vi "11c-async.vi"() -> ()   [LabVIEW 2018, in "LV2Julia_examples.lvlib"]
uses:
  LV2Julia_core/VIs/Server or client state.ctl
  LV2Julia_core/VIs/detailed error info.ctl
  LV2Julia_core/VIs/StackFrame.ctl
  LV2Julia_core/VIs/Commands.ctl
  be4745b6-8471-45fc-b8a0-8968ce92ea4b.vi
  877f6708-f4bd-42a3-8abe-32eb8c2c970e.vi
  be4745b6-8471-45fc-b8a0-8968ce92ea4b.vi/01ce1741-ea78-47f8-98ed-e79163fb1a9b.vi
  877f6708-f4bd-42a3-8abe-32eb8c2c970e.vi/896d20f1-cb1d-4420-8f1f-f93355f5adea.vi
  be4745b6-8471-45fc-b8a0-8968ce92ea4b.vi/01ce1741-ea78-47f8-98ed-e79163fb1a9b.vi/cc3cf2af-bc3b-4fb6-855b-7562c4d0bfeb.vi
  be4745b6-8471-45fc-b8a0-8968ce92ea4b.vi/01ce1741-ea78-47f8-98ed-e79163fb1a9b.vi/c77cecd8-10de-4d46-bc1c-57302a887fda.vi
  be4745b6-8471-45fc-b8a0-8968ce92ea4b.vi/01ce1741-ea78-47f8-98ed-e79163fb1a9b.vi/2cafb1dd-d397-4b79-911a-06d102936120.vi
  877f6708-f4bd-42a3-8abe-32eb8c2c970e.vi/896d20f1-cb1d-4420-8f1f-f93355f5adea.vi/9892c125-836d-426b-b144-8af50d50507b.vi
  877f6708-f4bd-42a3-8abe-32eb8c2c970e.vi/896d20f1-cb1d-4420-8f1f-f93355f5adea.vi/80aac079-9052-42cf-b2c3-c29da6bba58d.vi
  877f6708-f4bd-42a3-8abe-32eb8c2c970e.vi/896d20f1-cb1d-4420-8f1f-f93355f5adea.vi/6d5e1d21-cb4d-4981-8d16-85d9352ac501.vi
  LV2Julia_core/VIs/jl-scripts path.vi
  LV2Julia_core/VIs/check ID validity.vi
  LV2Julia_core/VIs/bindata_descr to JSON.vi
  LV2Julia_core/VIs/check cluster field names.vi
  LV2Julia_core/VIs/concat JSON.vi
  LV2Julia_core/VIs/build request.vi
  LV2Julia_core/VIs/Parse server response.vi
  LV2Julia_core/VIs/log jl exceptions.vi
  LV2Julia_examples.lvlib
  LV2Julia_core/LV2Julia_core.lvlib
panel:
  in  "Timeout (s)":dbl
  out "notif 2":bool
  out "Boolean":bool
  out "notification":bool
  in  "stop polling":bool
  out "stopping":bool
  out "done":bool
  out "ticket":i32
  in  "summands":cluster{"x":dbl, "y":dbl}={"x"=2.0, "y"=2.0}
  in  "next":bool
  out "x+y":dbl=nan
  out "detailed error info":T1
  out "current error":errorcluster
  out "final error":errorcluster
  out "short err code":u8
  in  "stop":bool
  out "ZMQ timeout":bool
  out "Julia script file path":path
  out "temporary script path":path
  out "Jl Server state":T3
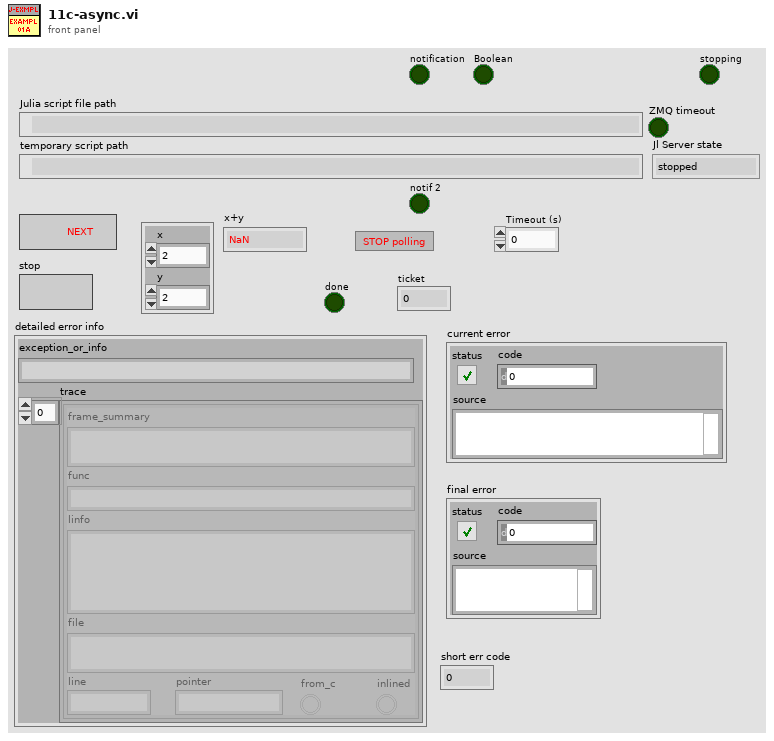
[diagram p1: front panel]
types:
  T1 = typedef "LV2Julia_core.lvlib/detailed error info.ctl" = cluster{"exception_or_info":string, "trace":T2[]}
  T2 = typedef "LV2Julia_core.lvlib/StackFrame.ctl" = cluster{"frame_summary":string, "func":string, "linfo":string, "file":string, "line":i32, "pointer":u64, "from_c":bool, "inlined":bool}
  T3 = typedef "LV2Julia_core.lvlib/Server or client state.ctl" = enum16{"stopped", "running", "unknown"}
  T4 = typedef "LV2Julia_core.lvlib/Commands.ctl" = enum16{"Start Jl-server & Init LV-client", "Send request & Get response ", "Stop Jl-server & Cleanup LV-client", "Cleanup LV-client", "Start Jl-server", "Stop Jl-server", "Init LV-Client", "Cleanup LV-Client", "(not allowed)", "Set LV Client state", "Set Jl Server state", "set ZMQ timeout", "read ZMQ timeout", "read-out state"}
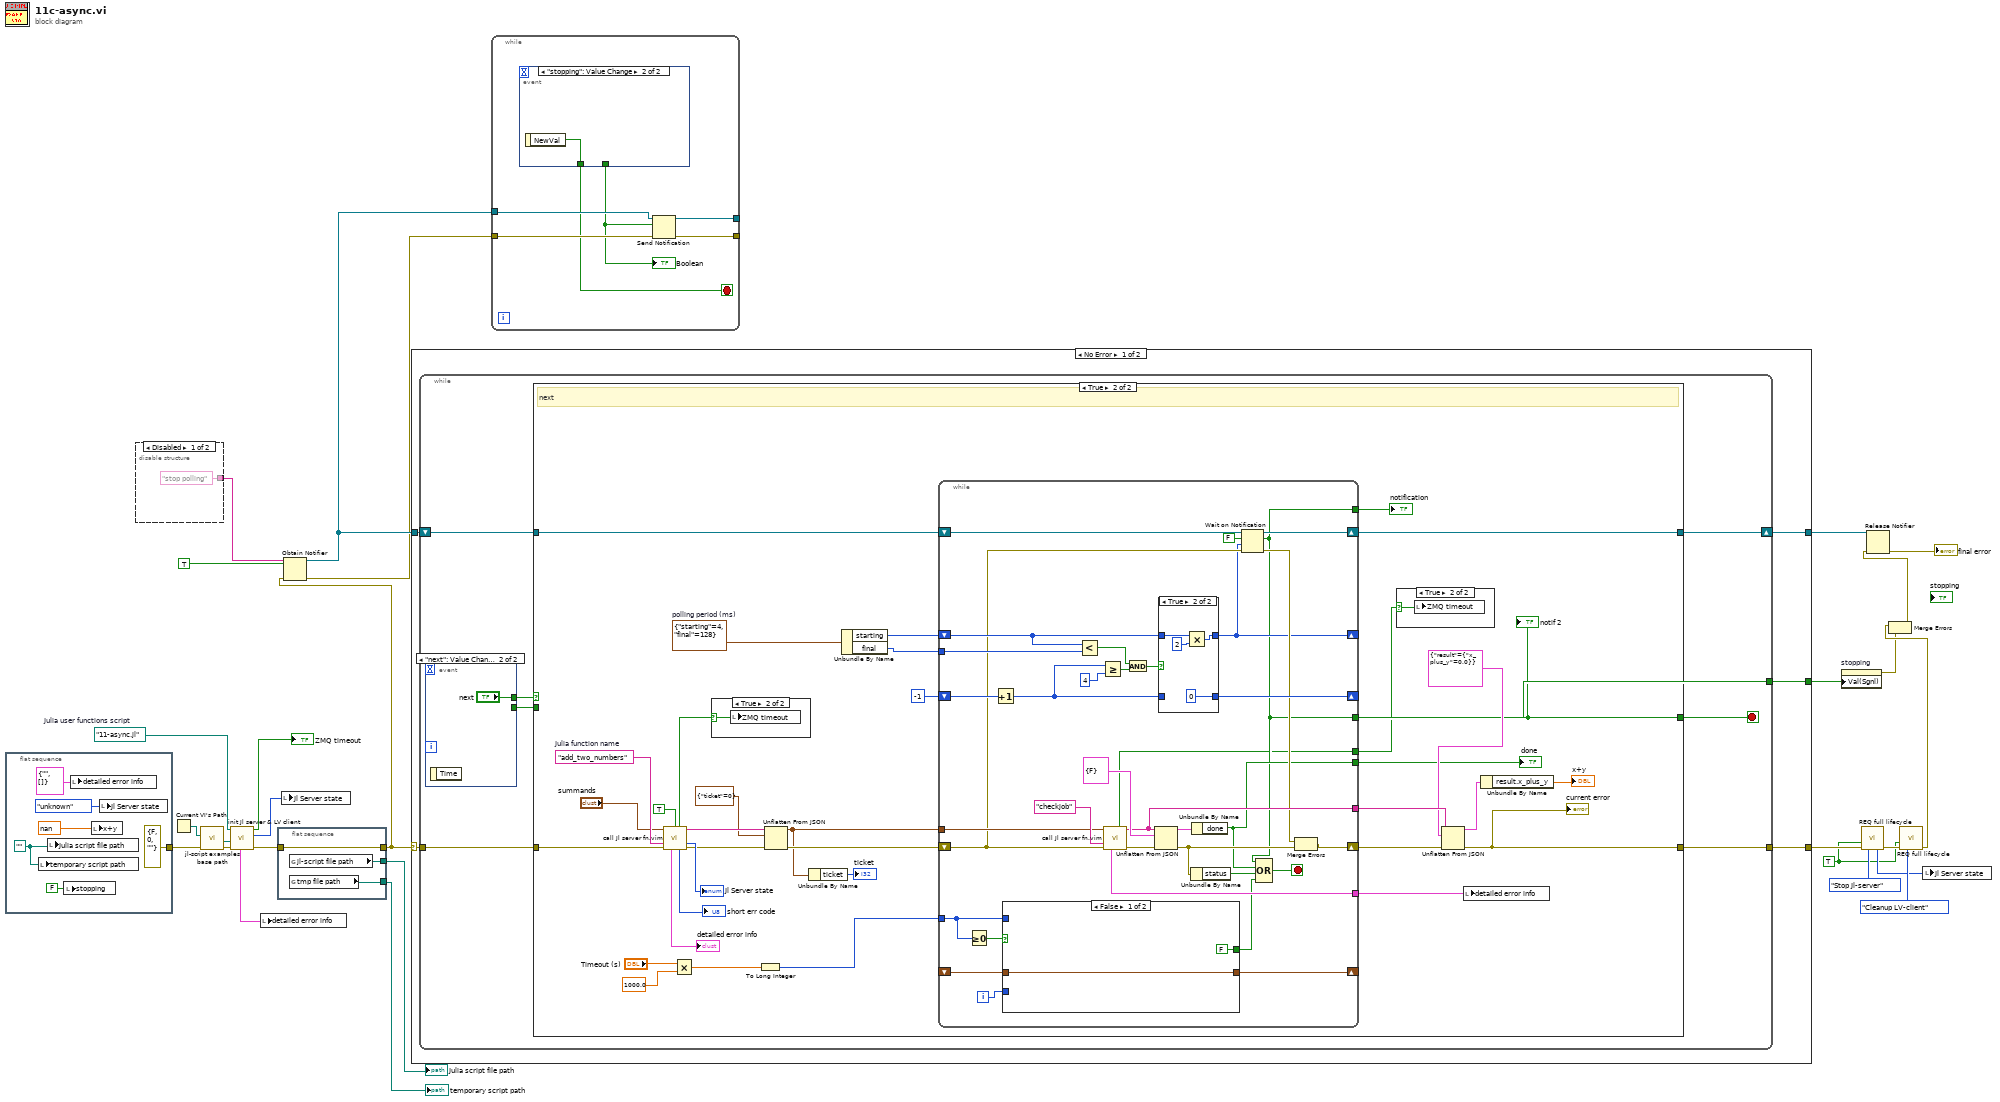
[diagram p0: block diagram]
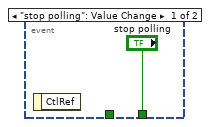
[diagram p3: hidden frame]
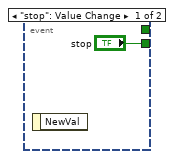
[diagram p4: hidden frame]
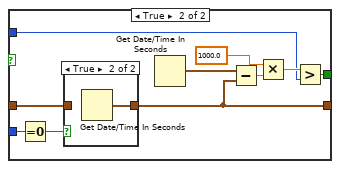
[diagram p7: hidden frame]
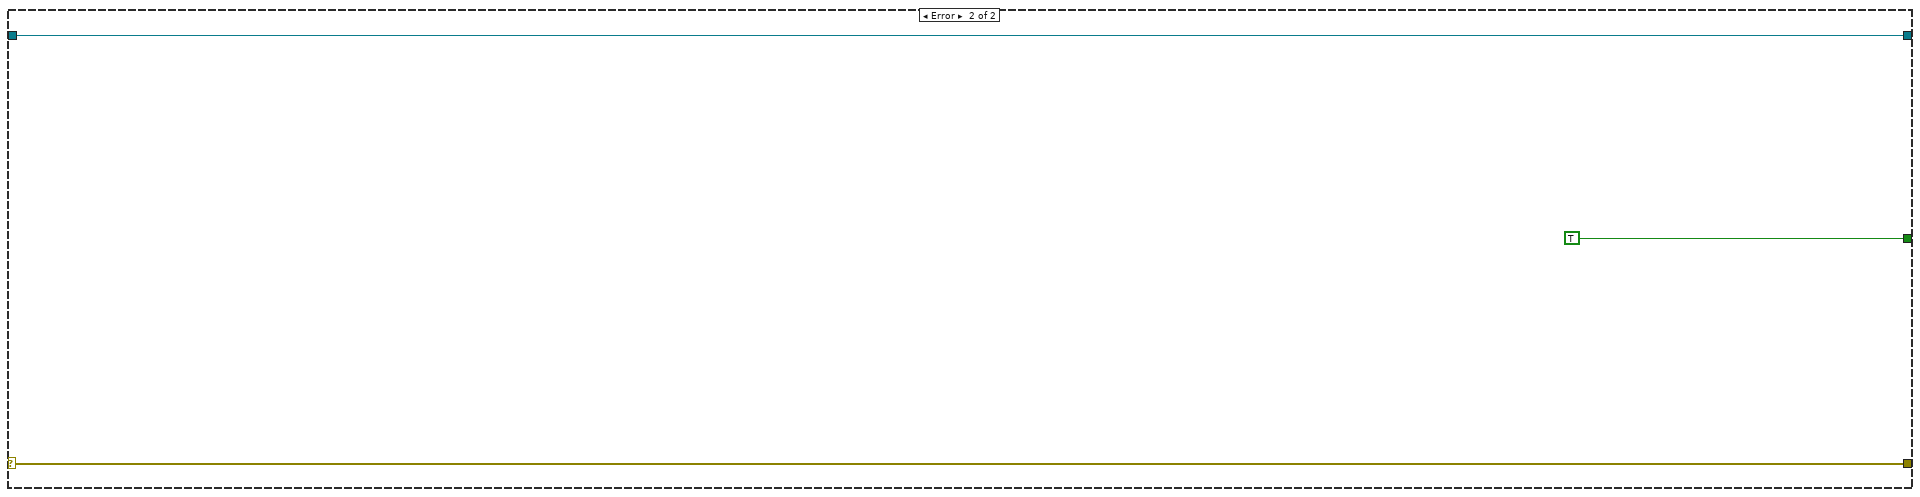
[diagram p11: hidden frame]
diagram:
  w21 = path "11-async.jl"  # Julia user functions script
  w5 = TRUE ("Force command")
  n1 = flat-sequence {
    tunnel: [errorcluster {"status"=FALSE, "code"=0, "source"=""} ("error in (no error)")] -> w17
    frame #0 {
      w30 = path ""
      n2 = local write "temporary script path"(w30) -> ()
      n3 = local write "Julia script file path"(w30) -> ()
      n4 = local write "stopping"(FALSE ("stopping")) -> ()
      n5 = local write "detailed error info"(T1 {"exception_or_info"="", "trace"=[]} ("detailed error info")) -> ()
      n6 = local write "x+y"(nan ("Server response")) -> ()
      n7 = local write "Jl Server state"(Server_or_client_state."unknown" ("Jl Server state out")) -> ()
    }
  }
  n8 = disable-structure shown="Disabled" {
    disable-tunnel: ["stop polling" ("name (unnamed)") _] -> w11
    frame Disabled {
    }
    frame Enabled {
    }
  }
  n9 = Current VI's Path() -> (path=w14:path)
  n10 = call "jl-script examples base path.vi"("error in (no error)"=w17, "calling example VI path"=w14) -> ("error out"=w16:errorcluster, "jl-script-examples base path"=w15:path)  [unwired: 8 in]
  n11 = call "init Jl server & LV client.vi"("error in (no error)"=w16, "Base path (not a path)"=w15, "Julia user functions script"=w21) -> ("error out"=w19:errorcluster, "Jl Server state out"=w18:T3, "timeout?"=→"ZMQ timeout":bool, "detailed error info"=w13:T1)  [unwired: 3 in, 2 out]
  n12 = local write "detailed error info"(w13) -> ()
  n13 = flat-sequence {
    tunnel: [w38] -> w9
    tunnel: w19 -> [w38]
    tunnel: [w37] -> w23
    tunnel: [w36] -> w24
    frame #0 {
      n14 = global read "jl-scripts path.vi" "jl-script file path"() -> (w37:path)
      n15 = global read "jl-scripts path.vi" "tmp file path"() -> (w36:path)
    }
  }
  n16 = local write "Jl Server state"(w18) -> ()
  n17 = Obtain Notifier(name (unnamed)=w11, notification data type=TRUE, error in (no error)=w9) -> (notifier out=w10:refnum<notifier>, error out=w8:errorcluster)  [unwired: 1 in, 1 out]
  n18 = case shown="No Error" w9 {
    selector: w9 -> [w42 w150]
    tunnel: [w43 w150] -> w28
    tunnel: w10 -> [w41 w149]
    tunnel: [w40 w149] -> w7
    tunnel: [w39 TRUE ("stop")] -> w1
    frame No Error {
      n19 = while {
        tunnel: w42 -> [w49]
        tunnel: [w50] -> w43
        shift-right: [w45] -> w40
        shift-left: w41 -> [w46]
        tunnel: [w44] -> w39
        stop <- w44 stop-if-true
        n20 = event shown="[1] \"next\": Value Change" {
          selector: _ -> [_ _]
          dyn-events: _ -> [_ _]
          timeout: _ -> [_ _]
          tunnel: [_ "next"] -> w48
          tunnel: ["stop" _] -> w47
          event "stop": Value Change {
            n21 = event-data() -> ()  [unwired: 1 in, 1 out]
          }
          event "next": Value Change {
            n22 = event-data() -> ()  [unwired: 1 in, 1 out]
          }
        }
        n23 = case shown="True" w48 {
          tunnel: [w53 w81] -> w50
          tunnel: w49 -> [w53 w83]
          tunnel: [w54 w64] -> w44
          tunnel: w47 -> [w54 _]
          tunnel: w46 -> [w55 w66]
          tunnel: [w55 w65] -> w45
          frame False {
            # "stop"
          }
          frame True {
            w70 = cluster{"starting":i32, "final":i32} {"starting"=4, "final"=128}  # polling period (ms)
            w89 = "add_two_numbers"  # Julia function name
            # "next"
            n24 = call "call Jl server fn.vim"("Arguments 1"="summands", "async call (false)"=TRUE ("timeout?"), "fun2call"=w89, "error in (no error)"=w83) -> ("timeout?"=w86:bool, "JSON received"=w79:string, "Jl Server state out"=→"Jl Server state":T3, "detailed error info"=→"detailed error info":T1, "return code"=→"short err code":u8, "error out"=w78:errorcluster)  [unwired: 5 in, 1 out]
            n25 = Multiply(x="Timeout (s)", y=1000.0) -> (x*y=w61:dbl)
            n26 = case shown="True" w86 {
              selector: w86 -> [_ w147]
              frame False {
              }
              frame True {
                n27 = local write "ZMQ timeout"(w147) -> ()
              }
            }
            n28 = To Long Integer(number=w61) -> (32bit integer=w60:i32)
            n29 = Unflatten From JSON(JSON string=w79, type and defaults=cluster{"ticket":i32} {"ticket"=0} ("parsed response"), error in (no error)=w78) -> (value=w75:cluster{"ticket":i32}, error out=w76:errorcluster)  [unwired: 4 in]
            n30 = Unbundle By Name(w75) -> ("ticket"=→"ticket":i32)
            n31 = Unbundle By Name(w70) -> ("starting"=w69:i32, "final"=w67:i32)
            n32 = while {
              tunnel: w75 -> [w125]
              tunnel: [w121] -> w73
              shift-right: [w106] -> w72
              shift-left: w76 -> [w107]
              shift-right: [w103] -> _
              shift-left: w69 -> [w111]
              shift-right: [w116] -> _
              shift-left: -1 ("counter") -> [w117]
              tunnel: w67 -> [w113]
              shift-right: [w104] -> w65
              shift-left: w66 -> [w108]
              tunnel: [w95] -> w64
              tunnel: w60 -> [w92]
              shift-right: [w97] -> _
              shift-left: _ -> [w100]
              tunnel: [w99] -> w59
              tunnel: [w98] -> w58
              tunnel: [w95] -> w57
              tunnel: [w94] -> w56
              i -> [w101]
              stop <- w119 stop-if-true
              n33 = Greater Or Equal To 0?(x=w92) -> (x >= 0?=w93:bool)
              n34 = Increment(x=w117) -> (x+1=w110:i32)
              n35 = case shown="False" w93 {
                tunnel: w101 -> [_ w138]
                tunnel: w100 -> [w128 w136]
                tunnel: [w128 w134] -> w97
                tunnel: w92 -> [_ w130]
                tunnel: [FALSE w129] -> w96
                frame False {
                }
                frame True {
                  n36 = Equal To 0?(x=w138) -> (x = 0?=w137:bool)
                  n37 = case shown="True" w137 {
                    tunnel: [w139 w140] -> w134
                    tunnel: w136 -> [w139 _]
                    frame False {
                    }
                    frame True {
                      n38 = Get Date/Time In Seconds() -> (seconds since 1Jan1904=w140:timestamp)
                    }
                  }
                  n39 = Get Date/Time In Seconds() -> (seconds since 1Jan1904=w135:timestamp)
                  n40 = Subtract(x=w135, y=w134) -> (x-y=w133:dbl)
                  n41 = Multiply(x=1000.0, y=w133) -> (x*y=w131:dbl)
                  n42 = Greater?(x=w131, y=w130) -> (0:w129:bool)
                }
              }
              n43 = Less?(x=w111, y=w113) -> (x < y?=w112:bool)
              n44 = Greater Or Equal?(x=w110, y=4) -> (x >= y?=w114:bool)
              n45 = call "call Jl server fn.vim"("Arguments 1"=w125, "fun2call"="checkjob" ("Julia function name"), "error in (no error)"=w107) -> ("timeout?"=w94:bool, "JSON received"=w121:string, "detailed error info"=w98:T1, "error out"=w124:errorcluster)  [unwired: 6 in, 3 out]
              n46 = And(x=w112, y=w114) -> (x .and. y?=w109:bool)
              n47 = Unflatten From JSON(JSON string=w121, type and defaults=cluster{"done":bool} {"done"=FALSE}, error in (no error)=w124) -> (value=w122:cluster{"done":bool}, error out=w120:errorcluster)  [unwired: 4 in]
              n48 = case shown="True" w109 {
                tunnel: w110 -> [w142 _]
                tunnel: [w142 0] -> w116
                tunnel: w111 -> [w141 w145]
                tunnel: [w141 w144] -> w103
                frame False {
                }
                frame True {
                  n49 = Multiply(x=w145, y=2) -> (x*y=w144:i32)
                }
              }
              n50 = Unbundle By Name(w120) -> ("status"=w118:bool)
              n51 = Unbundle By Name(w122) -> ("done"=w99:bool)
              n52 = Wait on Notification(notifier=w108, ignore previous (F)=FALSE, timeout in ms (-1)=w103, error in (no error)=w107) -> (notifier out=w104:refnum<notifier>, notification=w95:bool, error out=w105:errorcluster)  [unwired: 1 out]
              n53 = Compound Arithmetic op=OR(w95, w99, w118, w96) -> (w119:bool)
              n54 = Merge Errors(w105, w120) -> (w106:errorcluster)
            }
            "notif 2" <- w64
            "done" <- w59
            "notification" <- w57
            n55 = case shown="True" w56 {
              selector: w56 -> [_ w91]
              frame False {
              }
              frame True {
                n56 = local write "ZMQ timeout"(w91) -> ()
              }
            }
            n57 = Unflatten From JSON(JSON string=w73, type and defaults=cluster{"result":cluster{"x_plus_y":dbl}} {"result"={"x_plus_y"=0.0}}, error in (no error)=w72) -> (value=w82:cluster{"result":cluster{"x_plus_y":dbl}}, error out=w81:errorcluster)  [unwired: 4 in]
            "current error" <- w81
            n58 = local write "detailed error info"(w58) -> ()
            n59 = Unbundle By Name(w82) -> ("result.x_plus_y"=→"x+y":dbl)
          }
        }
      }
    }
    frame Error {
    }
  }
  n60 = while {
    tunnel: w10 -> [w156]
    tunnel: [w155] -> _
    tunnel: w8 -> [w154]
    tunnel: [w153] -> _
    stop <- w151 stop-if-true
    n61 = event shown="[1] \"stopping\": Value Change" {
      selector: _ -> [_ _]
      dyn-events: _ -> [_ _]
      timeout: _ -> [_ _]
      tunnel: ["stop polling" _] -> w152
      tunnel: [_ w158] -> w151
      event "stop polling": Value Change {
        n62 = event-data() -> ()  [unwired: 1 in, 1 out]
      }
      event "stopping": Value Change {
        n63 = event-data() -> ("NewVal"=w158:bool)  [unwired: 1 in]
      }
    }
    "Boolean" <- w152
    n64 = Send Notification(notification=w152, notifier=w156, error in (no error)=w154) -> (notifier out=w155:refnum<notifier>, error out=w153:errorcluster)
  }
  n65 = property on="stopping" class="Bool (strict)"("Val(Sgnl)"=w1) -> (error out=w2:errorcluster)  [unwired: 2 in, 1 out]
  n66 = call "REQ full lifecycle.vi"("Force command"=w5, "error in"=w28, "command"=Commands."Stop Jl-server") -> ("Jl Server state out"=w22:T3, "error out"=w26:errorcluster)  [unwired: 6 in, 5 out]
  n67 = call "REQ full lifecycle.vi"("Force command"=w5, "error in"=w26, "command"=Commands."Cleanup LV-client") -> ("error out"=w4:errorcluster)  [unwired: 6 in, 6 out]
  n68 = Merge Errors(w4, w2) -> (w3:errorcluster)
  n69 = Release Notifier(notifier=w7, error in (no error)=w3) -> (error out=→"final error":errorcluster)  [unwired: 1 in, 2 out]
  n70 = local write "Jl Server state"(w22) -> ()
  "temporary script path" <- w24
  "Julia script file path" <- w23
